vi "Register gRPC Methods.vi"(8 "error in (no error)":errorcluster, 11 "Template Server in":refnum<class "Query Server.lvclass">) -> (0 "error out":errorcluster, 3 "Template Server out":refnum<class "Query Server.lvclass">)   [LabVIEW 2019, in "Query Server.lvlib" / "Query Server.lvclass"]
uses:
  Query Server.lvclass
  typeDefs/Server gRPC UEs.ctl
  gRPC lvSupport/Server API/typeDefs/grpcId.ctl
  gRPC lvSupport/gprc-lvsupport.lvlib
  gRPC lvSupport/Server API/typeDefs/Generic Method Event Data.ctl
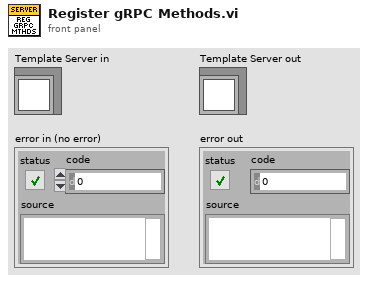
[diagram p1: front panel]
types:
  T1 = typedef "Query Server.lvlib/Query Server.lvclass/Server gRPC UEs.ctl" = cluster{"Generic Method Event":refnum<user-event>}
  T2 = typedef "Query Server.lvlib/gprc-lvsupport.lvlib/grpcId.ctl" = u64
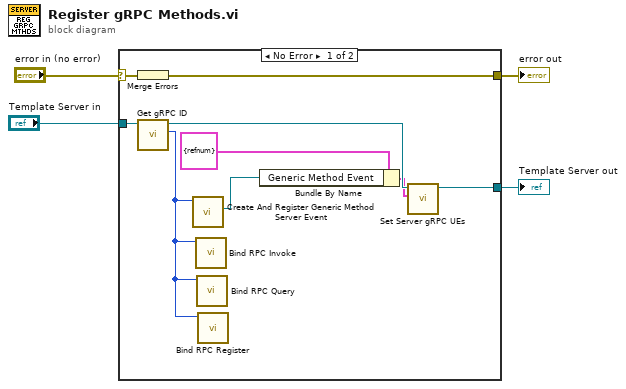
[diagram p0: block diagram]
diagram:
  n1 = case shown="No Error" "error in (no error)" {
    selector: "error in (no error)" -> [w8 w14]
    tunnel: "Template Server in" -> [w12 w15]
    tunnel: [w11 w14] -> w3
    tunnel: [w7 w15] -> w2
    frame No Error {
      n2 = Merge Errors(w8) -> (w11:errorcluster)
      n3 = call "Get gRPC ID.vi"("OOP Server in"=w12) -> ("gRPC ID"=w5:T2, "OOP Server out"=w13:refnum<class "Query Server.lvclass">)  [unwired: 9 in]
      n4 = call "Create And Register Generic Method Server Event.vi"("gRPCid server in"=w5) -> ("Generic Method Event"=w6:refnum<user-event>)  [unwired: 8 in, 2 out]
      n5 = call "Bind RPC Invoke.vi"("gRPCid server in"=w5) -> ()  [unwired: 7 in, 4 out]
      n6 = call "Bind RPC Query.vi"("gRPCid server in"=w5) -> ()  [unwired: 7 in, 4 out]
      n7 = call "Bind RPC Register.vi"("gRPCid server in"=w5) -> ()  [unwired: 7 in, 4 out]
      n8 = Bundle By Name ("Bundle gRPC UEs")(cluster=T1 {"Generic Method Event"=refnum} ("gRPC Server Method Events"), "Generic Method Event"=w6) -> (w10:T1)
      n9 = call "Set Server gRPC UEs.vi"("Server gRPC UEs"=w10, "OOP Server in"=w13) -> ("OOP Server out"=w7:refnum<class "Query Server.lvclass">)  [unwired: 9 in]
    }
    frame Error {
    }
  }
  "error out" <- w3
  "Template Server out" <- w2
